vi "util_launch_manual_action.vi"(5 "waitgroup":T1, 7 "change_in_event":refnum<user-event>, 8 "error in (no error)":errorcluster, 10 "data":variant, 11 "vi_reference":variant) -> (0 "error out":errorcluster)   [LabVIEW 2015, in "lv-recipe-machine.lvlib"]
uses:
  lv-recipe-machine.lvlib
  <userlib>/antonio-alexander/lv-waitgroup/public/_controls/api_waitgroup.ctl
  public/_controls/change.ctl
  public/_controls/vi_reference_manual_action.ctl
  <userlib>/antonio-alexander/lv-waitgroup/lv-waitgroup.lvlib
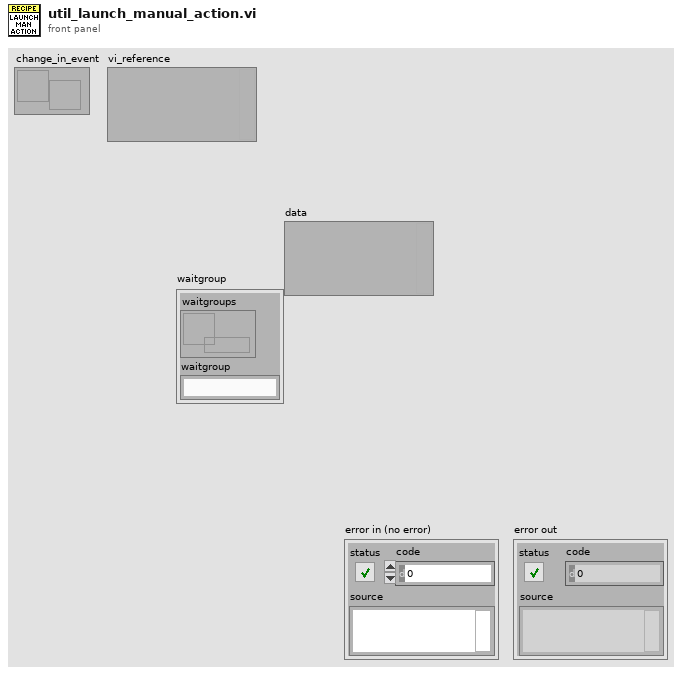
[diagram p1: front panel]
types:
  T1 = typedef "lv-waitgroup.lvlib/api_waitgroup.ctl" = cluster{"waitgroups":refnum<data-value>, "waitgroup":string}
  T2 = typedef "lv-recipe-machine.lvlib/vi_reference_manual_action.ctl" = refnum<vi>
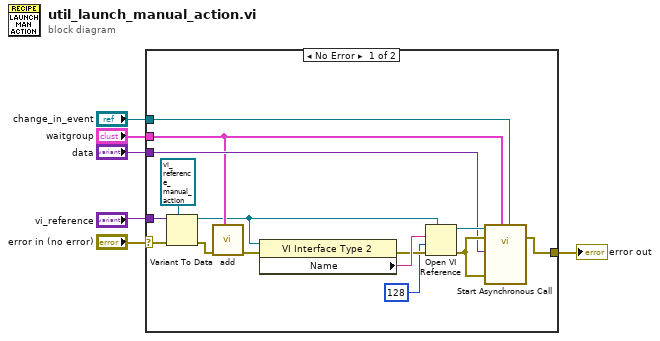
[diagram p0: block diagram]
diagram:
  n1 = case shown="No Error" "error in (no error)" {
    selector: "error in (no error)" -> [w9 w22]
    tunnel: "waitgroup" -> [w13 _]
    tunnel: [w15 w22] -> w4
    tunnel: "data" -> [w14 _]
    tunnel: "change_in_event" -> [w12 _]
    tunnel: "vi_reference" -> [w7 _]
    frame No Error {
      n2 = Variant To Data(error in=w9, type=T2 refnum ("step_vi_reference"), Variant=w7) -> (data=w10:T2, error out=w8:errorcluster)
      n3 = call <userlib>:"add.vi"("waitgroup"=w13, "error in (no error)"=w8) -> ("error out"=w20:errorcluster)  [unwired: 9 in]
      n4 = property class="VI Interface Type 2"(reference=w10, error in=w20) -> (error out=w18:errorcluster, "Name"=w19:string)  [unwired: 1 out]
      n5 = Open VI Reference(type specifier VI Refnum (for type only)=w10, vi path=w19, options=128, error in (no error)=w18) -> (vi reference=w17:T2, error out=w21:errorcluster)  [unwired: 2 in]
      n6 = call-by-ref "Start Asynchronous Call"(reference=w17, error in=w21, "change_in_event"=w12, "waitgroup"=w13, 8:"error in (no error)"=w21, "data"=w14) -> (error out=w15:errorcluster)  [unwired: 7 in, 2 out]
    }
    frame Error {
    }
  }
  "error out" <- w4
